vi "Get Array Value at Index - 1D Array Boolean.vi"(6 "Return Default if Null? (T)":bool=TRUE, 8 "error in (no error)":errorcluster, 9 "Default Value if JSON Null":bool[](array[boolean]), 10 "Index":i32, 11 "JSON Tree In (JSON Array)":variant) -> (0 "error out":errorcluster, 1 "is JSON Null?":bool, 2 "1D Boolean Array Value":bool[](array[boolean]), 3 "JSON Tree Out Passthrough":variant)   [LabVIEW 2011, in "i3-json.lvlib"]
doc: "Use this template to build a VI to use as a subVI."
uses:
  i3-json.lvlib
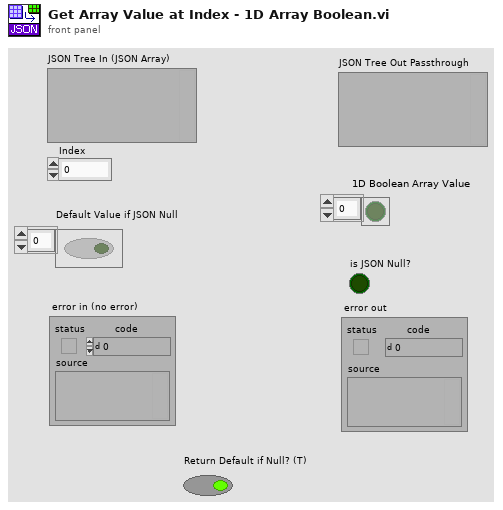
[diagram p1: front panel]
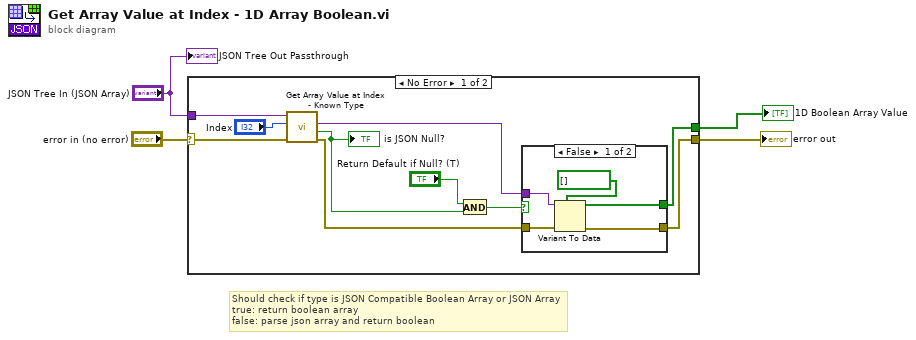
[diagram p0: block diagram]
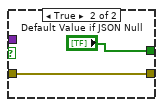
[diagram p2: hidden frame]
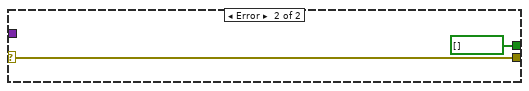
[diagram p3: hidden frame]
diagram:
  # "Should check if type is JSON Compatible Boolean Array or JSON Array\ntrue: return boolean array\nfalse: parse json array and return boolean"
  n1 = case shown="No Error" "error in (no error)" {
    selector: "error in (no error)" -> [w12 w23]
    tunnel: [w8 w23] -> w3
    tunnel: "JSON Tree In (JSON Array)" -> [w14 _]
    tunnel: [w5 bool[] [] ("Default Value if JSON Null")] -> w2
    frame No Error {
      n2 = call "Get Array Value at Index - Known Type.vi"("error in (no error)"=w12, "Index"="Index", "JSON Tree In (JSON Array)"=w14) -> ("error out"=w9:errorcluster, "is JSON Null?"=w6:bool, "Value"=w7:variant)  [unwired: 3 in, 3 out]
      "is JSON Null?" <- w6
      n3 = And(x="Return Default if Null? (T)", y=w6) -> (x .and. y?=w10:bool)
      n4 = case shown="False" w10 {
        tunnel: w9 -> [w19 w21]
        tunnel: [w16 w21] -> w8
        tunnel: w7 -> [w18 _]
        tunnel: [w17 "Default Value if JSON Null"] -> w5
        frame False {
          n5 = Variant To Data(error in=w19, type=bool[] [], Variant=w18) -> (data=w17:bool[], error out=w16:errorcluster)
        }
        frame True {
        }
      }
    }
    frame Error {
    }
  }
  "error out" <- w3
  "1D Boolean Array Value" <- w2
  "JSON Tree Out Passthrough" <- "JSON Tree In (JSON Array)"
